vi "lAUNCHER.vi"() -> ()   [LabVIEW 2020]
uses:
  UI Actor/UI Actor.lvclass
  C:/Program Files/National Instruments/LabVIEW 2020/vi.lib/ActorFramework/Actor/Actor.lvclass
  UI Actor/UI Actor.lvclass/UI Actor.ctl
  UI Actor/Write Coins.vi
  UI Actor/Write Productos .vi
  <vilib>/ActorFramework/Actor/Actor.lvclass
panel:
  in  "Productos":T1(ring)
  in  "Coins":enum16{"MNX", "Corona Islandesa"}(ring)
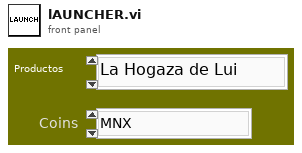
[diagram p1: front panel]
types:
  T1 = enum16{"La Hogaza de Lui", "MiniSuper Doña Rata"}
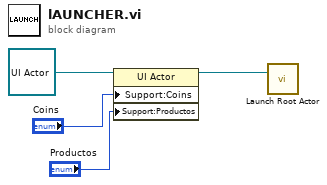
[diagram p0: block diagram]
diagram:
  n1 = property class="UI Actor"(reference=refnum<class "UI Actor.lvclass"> refnum ("UI Actor.lvlib:UI Actor.lvclass"), "Support:Coins"="Coins", "Support:Productos "="Productos") -> (reference out=w3:refnum<class "UI Actor.lvclass">)  [unwired: 1 in, 1 out]
  n2 = call <vilib>:"Launch Root Actor.vi"("Actor"=w3) -> ()  [unwired: 9 in, 2 out]
